vi "Write Single Register.vi"(8 "error in":errorcluster, 9 "register value":u16, 10 "address":u16, 11 "device data model in":refnum<class "Device Data Model.lvclass">) -> (0 "error out":errorcluster, 3 "device data model out":refnum<class "Device Data Model.lvclass">)   [LabVIEW 2014, in "MyLib.lvlib" / "Device Data Model.lvclass"]
doc: "Writes the value of a single holding register."
uses:
  Device Data Model.lvclass
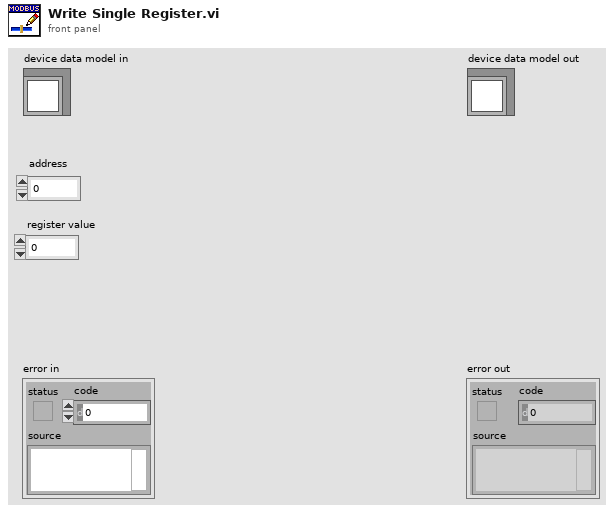
[diagram p1: front panel]
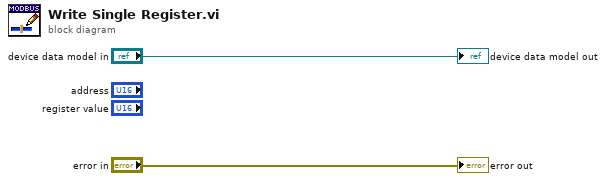
[diagram p0: block diagram]
diagram:
  "error out" <- "error in"
  "device data model out" <- "device data model in"
